vi "updateUnits.vi"(8 "error in (no error)":errorcluster, 11 "StaticOutputEditor in":refnum<class "StaticOutputEditor.lvclass">) -> (0 "error out":errorcluster, 3 "StaticOutputEditor out":refnum<class "StaticOutputEditor.lvclass">)   [LabVIEW 2011, in "Views.lvlib" / "ScriptEditor.lvlib" / "StaticOutputEditor.lvclass"]
uses:
  StaticOutputEditor.lvclass
  StaticOutputEditor.lvclass/StaticOutputEditor.ctl
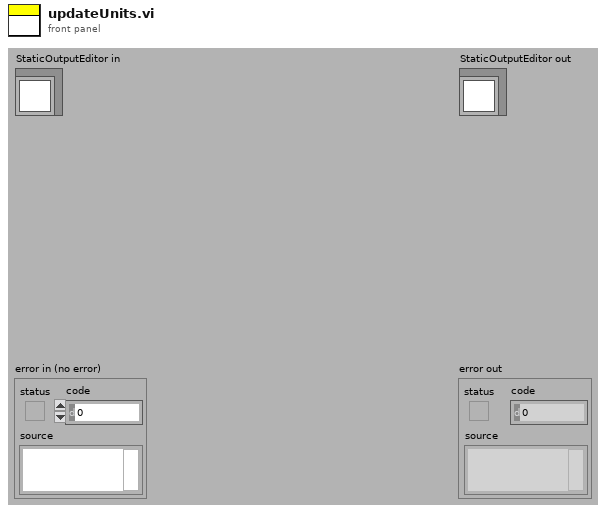
[diagram p1: front panel]
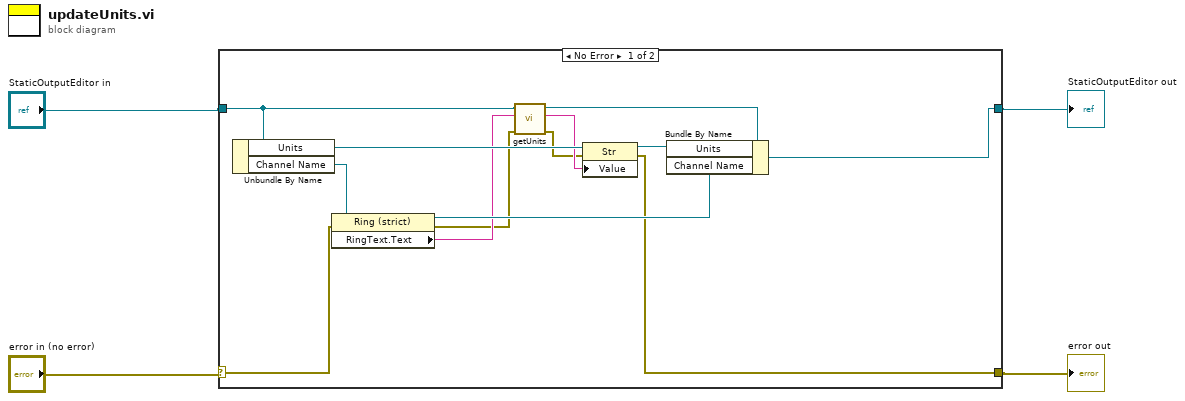
[diagram p0: block diagram]
diagram:
  n1 = case shown="No Error" "error in (no error)" {
    selector: "error in (no error)" -> [w11 w19]
    tunnel: [w5 w19] -> w1
    tunnel: [w6 w18] -> w2
    tunnel: "StaticOutputEditor in" -> [w14 w18]
    frame No Error {
      n2 = Unbundle By Name(w14) -> ("Units"=w15:refnum<vi>, "Channel Name"=w17:refnum<vi>)
      n3 = property class="Ring (strict)"(reference=w17, error in=w11) -> (reference out=w16:refnum<vi>, error out=w12:errorcluster, "RingText.Text"=w13:string)
      n4 = call "getUnits.vi"("error in (no error)"=w12, "channelName"=w13, "StaticOutputEditor in"=w14) -> ("error out"=w9:errorcluster, "units"=w10:string, "StaticOutputEditor out"=w7:refnum<class "StaticOutputEditor.lvclass">)  [unwired: 6 in]
      n5 = property class="Str"(reference=w15, error in=w9, "Value"=w10) -> (reference out=w8:refnum<vi>, error out=w5:errorcluster)
      n6 = Bundle By Name(cluster=w7, "Units"=w8, "Channel Name"=w16) -> (w6:refnum<class "StaticOutputEditor.lvclass">)
    }
    frame Error {
    }
  }
  "error out" <- w1
  "StaticOutputEditor out" <- w2
